vi "StartOperation (SubVI).vi"(8 "error in (no error)":errorcluster, 11 "Display Queue in":refnum<queue>) -> (0 "error out":errorcluster, 3 "Display Queue out":refnum<queue>)   [LabVIEW 2017]
doc: "Enqueues the appropiate commands to the Display Queue when a card is inserted into the ATM."
uses:
  Controls/DisplayControl.ctl
  Controls/DisplayCommand.ctl
  Controls/EnableDisableCommand.ctl
  Controls/UpdateMessageControl.ctl
  Controls/UpdateMessageCommand.ctl
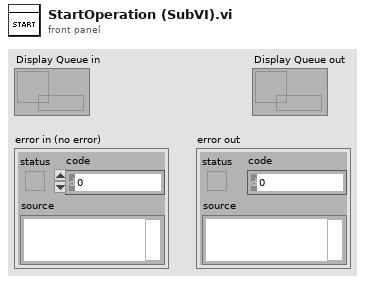
[diagram p1: front panel]
types:
  T1 = typedef "DisplayControl.ctl" = cluster{"Command":T2, "Data":variant}
  T2 = typedef "DisplayCommand.ctl" = enum16{"Initialize", "Open/Close Parcel", "Enable/Disable Controls", "FocusCursor", "UpdateMessage", "UpdateMenus", "FinishOperation", "Exit", "CleanUserInput"}
  T3 = typedef "UpdateMessageControl.ctl" = cluster{"Command":T4, "Data":variant}
  T4 = typedef "UpdateMessageCommand.ctl" = enum16{"SystemCrash2", "SystemCrash1", "Welcome", "MainMenu", "PhoneNumberFailed", "PhoneNumberSuccess", "ParcelNumberSuccess", "ParcelNumbertFailed", "SessionTerminate", "SessionFinished", "Deposit", "DepositComplete", "Withdrawal", "WithdrawalComplete", "WithdrawalFailed"}
  T5 = typedef "EnableDisableCommand.ctl" = enum16{"InitialSetup", "StartOperation", "EnableUserInput", "DisableUserInput", "EnableMenus", "DisableMenus"}
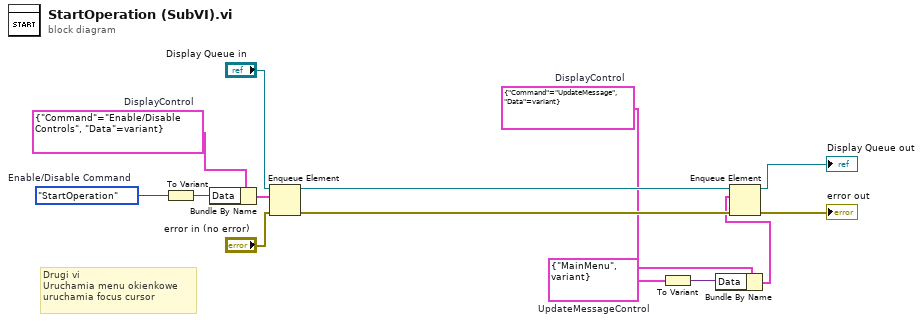
[diagram p0: block diagram]
diagram:
  w4 = T1 {"Command"=enum."UpdateMessage", "Data"=variant}  # DisplayControl
  w6 = T3 {"Command"=enum."MainMenu", "Data"=variant}  # UpdateMessageControl
  w13 = EnableDisableCommand."StartOperation"  # Enable/Disable Command
  w11 = T1 {"Command"=enum."Enable/Disable Controls", "Data"=variant}  # DisplayControl
  # "Drugi vi\nUruchamia menu okienkowe\nuruchamia focus cursor"
  n1 = To Variant(anything=w13) -> (Variant=w14:variant)
  n2 = Bundle By Name(cluster=w11, "Data"=w14) -> (w12:T1)
  n3 = Enqueue Element(queue="Display Queue in", element=w12, error in (no error)="error in (no error)") -> (queue out=w8:refnum<queue>, error out=w7:errorcluster)  [unwired: 1 in, 1 out]
  n4 = To Variant(anything=w6) -> (Variant=w5:variant)
  n5 = Bundle By Name(cluster=w4, "Data"=w5) -> (w3:T1)
  n6 = Enqueue Element(queue=w8, element=w3, error in (no error)=w7) -> (queue out=→"Display Queue out":refnum<queue>, error out=→"error out":errorcluster)  [unwired: 1 in, 1 out]
